vi "sendMultipleMessages.vi"(8 "error in (no error)":errorcluster {"code" format="Error %.0f"}, 9 "messageData":variant[](array[variant]), 10 "queueMessages":T2(array[cluster]), 11 "messageQueues":T1) -> (0 "error out":errorcluster {"code" format="Error %.0f"})   [LabVIEW 2017, in "Message Queue.lvlib"]
uses:
  Message Queue.lvlib
  messageQueues.ctl
  Message Cluster.ctl
  <vilib>/Utility/error.llb/Error Cluster From Error Code.vi
  <vilib>/ErrorRing/Error Ring.xnode
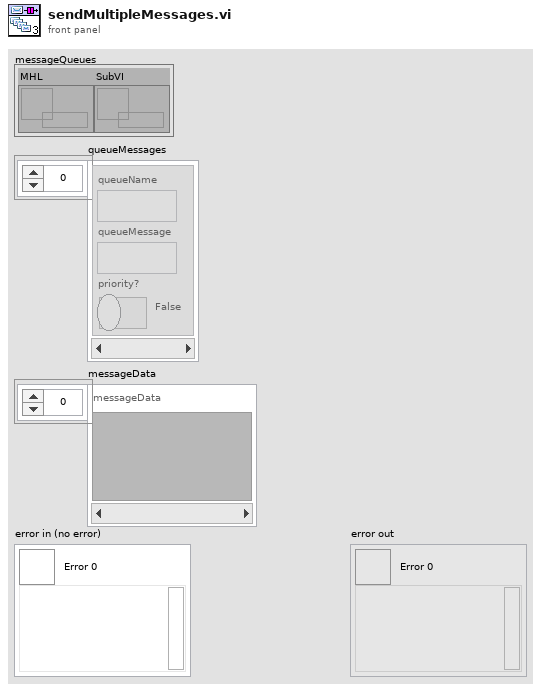
[diagram p1: front panel]
types:
  T1 = typedef "Message Queue.lvlib/messageQueues.ctl" = cluster{"MHL":refnum<queue>, "SubVI":refnum<queue>}
  T2 = cluster{"queueName":string, "queueMessage":string, "priority?":bool}[]
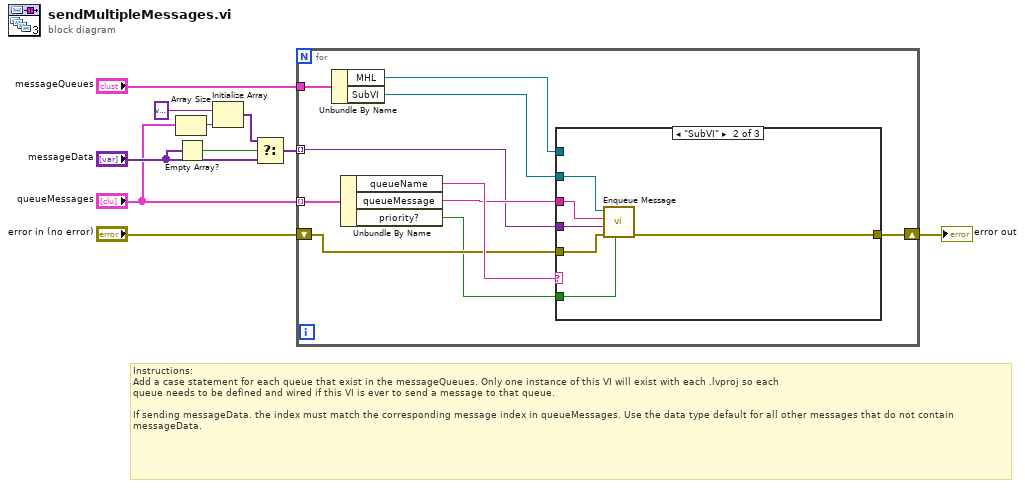
[diagram p0: block diagram]
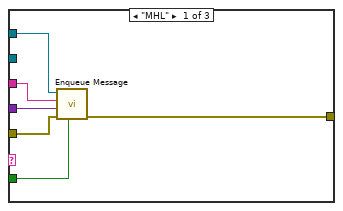
[diagram p2: hidden frame]
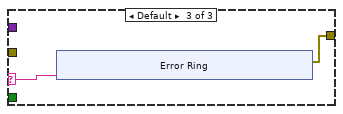
[diagram p3: hidden frame]
diagram:
  # "Instructions:\nAdd a case statement for each queue that exist in the messageQueues. Only one instance of this VI will exist with each .lvproj so each\nqueue needs to be defined and wired if this VI is ever to send a message to that queue.\n\nIf sending messageData. the index must match the corresponding message index in queueMessages. Use the data type default for all other messages that do not contain messageData."
  n1 = Array Size(array="queueMessages") -> (size(s)=w6:i32)
  n2 = Empty Array?(array="messageData") -> (empty?=w5:bool)
  n3 = Initialize Array(variant, w6) -> (w2:variant[])
  n4 = Select(t=w2, s=w5, f="messageData") -> (s? t:f=w3:variant[])
  n5 = for {
    tunnel: "queueMessages" -> [w20] mode=indexing
    shift-right: [w18] -> w10
    shift-left: "error in (no error)" -> [w17]
    tunnel: w3 -> [w12] mode=indexing
    tunnel: "messageQueues" -> [w15]
    n6 = Unbundle By Name(w15) -> ("MHL"=w13:refnum<queue>, "SubVI"=w14:refnum<queue>)
    n7 = Unbundle By Name(w20) -> ("queueName"=w19:string, "queueMessage"=w16:string, "priority?"=w11:bool)
    n8 = case shown="\"SubVI\"" w19 {
      selector: w19 -> [_ _ w34]
      tunnel: [w26 w32 w33] -> w18
      tunnel: w17 -> [w25 w31 _]
      tunnel: w16 -> [w24 w30 _]
      tunnel: w14 -> [_ w29 _]
      tunnel: w13 -> [w23 _ _]
      tunnel: w12 -> [w21 w28 _]
      tunnel: w11 -> [w22 w27 _]
      frame "MHL" {
        n9 = call "Enqueue Message.vi"("Priority Message? (F)"=w22, "error in (no error)"=w25, "Message Data"=w21, "Message"=w24, "Message Queue"=w23) -> ("error out"=w26:errorcluster)  [unwired: 5 in, 1 out]
      }
      frame "SubVI" {
        n10 = call "Enqueue Message.vi"("Priority Message? (F)"=w27, "error in (no error)"=w31, "Message Data"=w28, "Message"=w30, "Message Queue"=w29) -> ("error out"=w32:errorcluster)  [unwired: 5 in, 1 out]
      }
      frame Default {
        n11 = xnode "Error Ring"("parameter 0"=w34) -> ("error out"=w33:errorcluster)
      }
    }
  }
  "error out" <- w10
